vi "proptest_runtime class.vi"() -> (0 "error 538301":errorcluster, 2 "class name empty=ok":bool)   [LabVIEW 2025, in "NISE_CEF_Tests.lvlib"]
uses:
  NISE_CEF_Tests.lvlib
  Trunk/Configuration Framework/serializable configuration/NISE_CEF_serializable configuration.lvclass
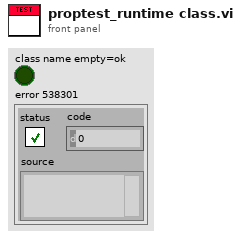
[diagram p1: front panel]
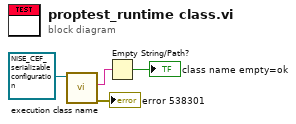
[diagram p0: block diagram]
diagram:
  n1 = call-dynamic "execution class name.vi"("configuration in"=refnum<class "NISE_CEF_serializable configuration.lvclass"> refnum ("configuration")) -> ("error out"=→"error 538301":errorcluster, "execution class"=w1:string)  [unwired: 8 in, 1 out]
  n2 = Empty String/Path?(string/path=w1) -> (empty?=→"class name empty=ok":bool)
